vi "QTrkQueueImageU8.vi"(0 "QTrk Instance":T1, 1 "frame":u32, 3 "zlutIndex":i32, 5 "error in (no error)":errorcluster, 7 "image":u8[][](array[numeric]), 11 "Timestamp":i32) -> (14 "QTrk Instance":T1, 19 "error out":errorcluster)   [LabVIEW 2011]
uses:
  QTrkInstance.ctl
  QTrkLocalizationJob.ctl
  XYZf.ctl
  QTrkDLL.vi
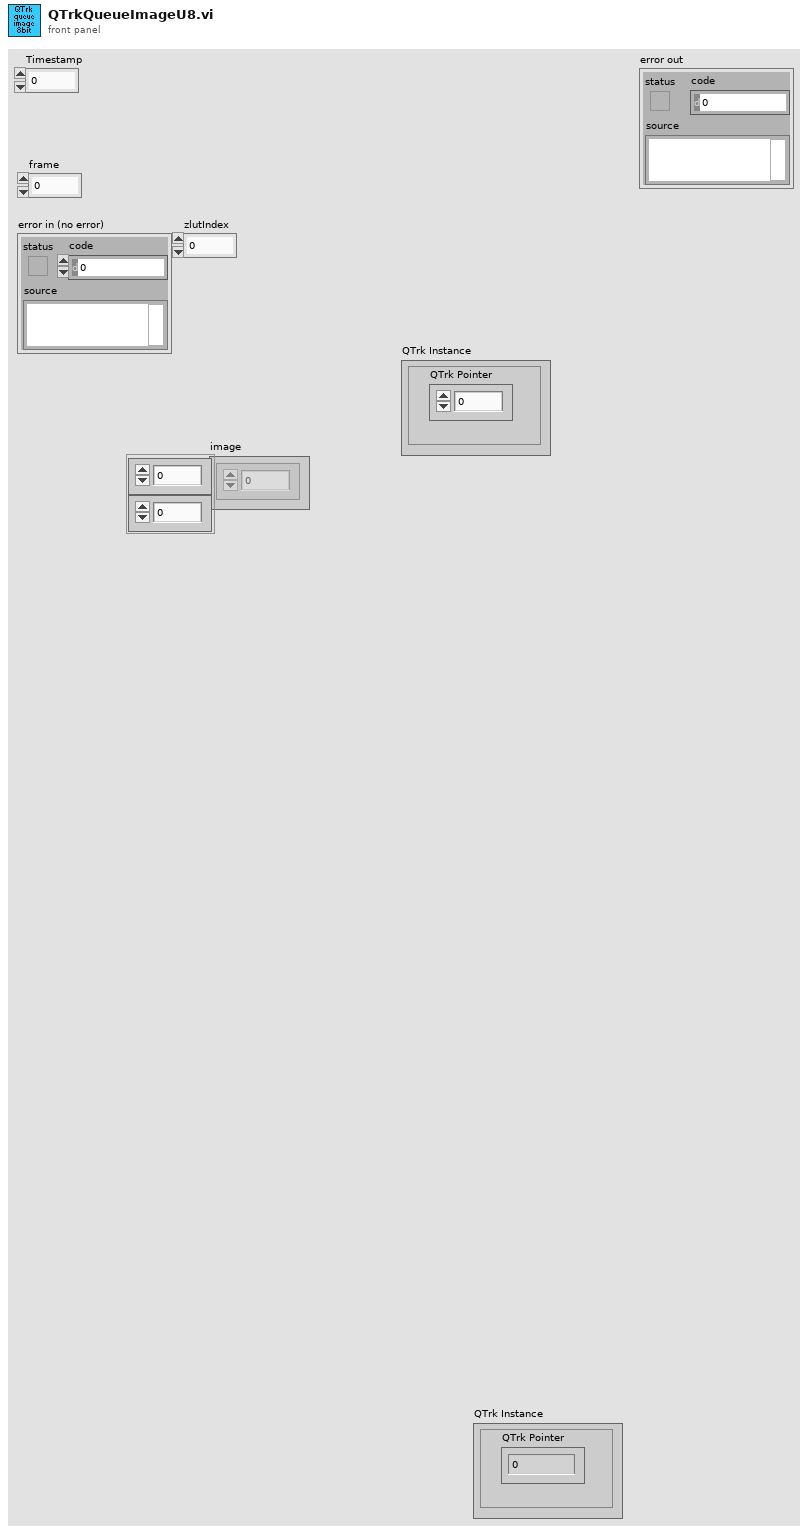
[diagram p1: front panel]
types:
  T1 = typedef "QTrkInstance.ctl" = cluster{"QTrk Pointer":u64}
  T2 = typedef "QTrkLocalizationJob.ctl" = cluster{"Frame#":u32, "Timestamp":u32, "ZLUT Index / bead#":i32, "Initial guess":T3}
  T3 = typedef "XYZf.ctl" = cluster{"X":sgl, "Y":sgl, "Z":sgl}
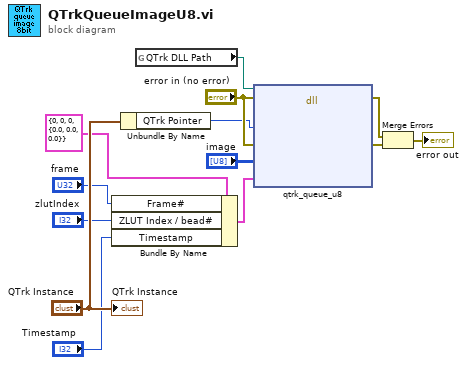
[diagram p0: block diagram]
diagram:
  n1 = Bundle By Name(cluster=T2 {"Frame#"=0, "Timestamp"=0, "ZLUT Index / bead#"=0, "Initial guess"={"X"=0.0, "Y"=0.0, "Z"=0.0}} ("Queue Params"), "Frame#"="frame", "ZLUT Index / bead#"="zlutIndex", "Timestamp"="Timestamp") -> (w4:T2)
  n2 = Unbundle By Name("QTrk Instance") -> ("QTrk Pointer"=w8:u64)
  n3 = global read "QTrkDLL.vi" "QTrk DLL Path"() -> (w12:path)
  n4 = dll-call lib="D:/jcnossen1/cudaqi-tracker/bin/jtrk-labview.dll" fn="qtrk_queue_u8"(path in=w12, error in="error in (no error)", "tracker"=w8, "error"="error in (no error)", "data"="image", "params"=w4) -> (error out=w9:errorcluster, "error"=w10:errorcluster)  [unwired: 5 in, 1 out]
  n5 = Merge Errors(w9, w10) -> (→"error out":errorcluster)
  "QTrk Instance" <- "QTrk Instance"
